vi "TrigBasicProps.vi"(0 "task in":refnum<k24>, 3 "error in (no error)":errorcluster) -> (1 "Slope":i32, 4 "PretriggerCount":i32, 5 "task out":refnum<k24>, 6 "DigLevel":i32, 7 "AnalogLevel":dbl, 8 "error out":errorcluster)   [LabVIEW 2010]
uses:
  C:/Program Files/National Instruments/LabVIEW 2010/vi.lib/ULx/ULx_LV.dll
  Program Files/National Instruments/LabVIEW 2010/vi.lib/ULx/ULx_LV.dll
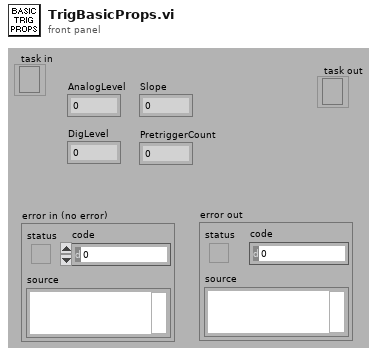
[diagram p1: front panel]
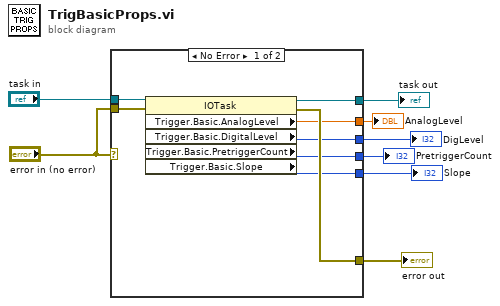
[diagram p0: block diagram]
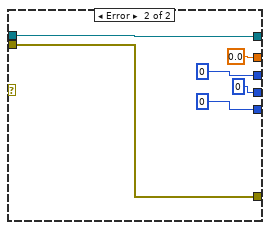
[diagram p2: hidden frame]
diagram:
  n1 = case shown="No Error" "error in (no error)" {
    tunnel: "task in" -> [w16 w22]
    tunnel: "error in (no error)" -> [w15 w21]
    tunnel: [w14 w22] -> w7
    tunnel: [w13 w21] -> w6
    tunnel: [w11 0 ("Trigger.Basic.Type")] -> w4
    tunnel: [w12 0.0 ("Trigger.Basic.AnalogLevel")] -> w3
    tunnel: [w10 0 ("Trigger.Basic.PretriggerCount")] -> w2
    tunnel: [w9 0 ("Trigger.Basic.Slope")] -> w1
    frame No Error {
      n2 = property class="IOTask"(reference=w16, error in=w15) -> (reference out=w14:refnum<k24>, error out=w13:errorcluster, "Trigger.Basic.AnalogLevel"=w12:dbl, "Trigger.Basic.DigitalLevel"=w11:i32, "Trigger.Basic.PretriggerCount"=w10:i32, "Trigger.Basic.Slope"=w9:i32)
    }
    frame Error {
    }
  }
  "task out" <- w7
  "error out" <- w6
  "DigLevel" <- w4
  "AnalogLevel" <- w3
  "PretriggerCount" <- w2
  "Slope" <- w1
